vi "Test GitHub Issues.vi"(8 "error in (no error)":errorcluster) -> (0 "error out":errorcluster)   [LabVIEW 2017]
uses:
  <vilib>/addons/_JKI Toolkits/Caraya/classes/Test/Test.lvclass
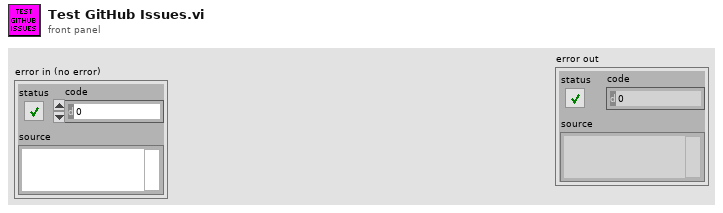
[diagram p1: front panel]
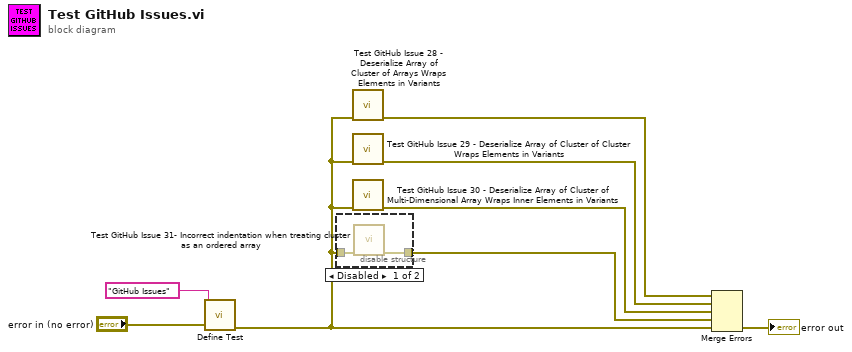
[diagram p0: block diagram]
diagram:
  n1 = call <vilib>:"Define Test.vi"("error in (no error)"="error in (no error)", "Label (VI Title)"="GitHub Issues") -> ("error out"=w2:errorcluster)  [unwired: 9 in]
  n2 = disable-structure shown="Disabled" {
    disable-tunnel: w2 -> [w10 _]
    disable-tunnel: [w9 _] -> w1
    frame Disabled {
      n3 = call "Test GitHub Issue 31- Incorrect indentation when treating cluster as an ordered array.vi"("error in (no error)"=w10) -> ("error out"=w9:errorcluster)  [unwired: 10 in]
    }
    frame Enabled {
    }
  }
  n4 = call "Test GitHub Issue 28 - Deserialize Array of Cluster of Arrays Wraps Elements in Variants.vi"("error in (no error)"=w2) -> ("error out"=w5:errorcluster)  [unwired: 10 in]
  n5 = call "Test GitHub Issue 29 - Deserialize Array of Cluster of Cluster Wraps Elements in Variants.vi"("error in (no error)"=w2) -> ("error out"=w4:errorcluster)  [unwired: 10 in]
  n6 = call "Test GitHub Issue 30 - Deserialize Array of Cluster of Multi-Dimensional Array Wraps Inner Elements in Variants.vi"("error in (no error)"=w2) -> ("error out"=w3:errorcluster)  [unwired: 10 in]
  n7 = Merge Errors(w5, w4, w3, w1, w2) -> (→"error out":errorcluster)
